vi "VITree.vi"   [LabVIEW 2016, in "DronaTest.lvlib"]
uses:
  DronaTest.lvlib
  APIs/Stimulus/ControlValue/typedef/Name&Occurrence.ctl
  APIs/Assert/AssertControlValue/AlmostEqual.vi
  APIs/Assert/AssertControlValue/Equal.vi
  APIs/Assert/AssertControlValue/NotEqual.vi
  APIs/Assert/AssertControlValue/Greater.vi
  APIs/Assert/AssertControlValue/GreaterOrEqual.vi
  APIs/Assert/AssertControlValue/Less.vi
  APIs/Assert/AssertControlValue/LessOrEqual.vi
  APIs/Assert/AssertControlValue/True.vi
  APIs/Assert/AssertControlValue/False.vi
  APIs/Assert/AssertControlDisable/AssertDisabled.vi
  APIs/Assert/AssertControlDisable/AssertDisabledAndGrayedOut.vi
  APIs/Assert/AssertControlDisable/AssertEnabled.vi
  APIs/Assert/AssertControlValue/Controls/Listbox/AssertValueByFocusIndex.vi
  APIs/Assert/AssertControlValue/Controls/Listbox/AssertValueByFocusName.vi
  APIs/Assert/AssertControlValue/Controls/Listbox/AssertValueByArrayIndex.vi
  APIs/Assert/AssertControlValue/Controls/Listbox/AssertValueByArrayName.vi
  APIs/Assert/AssertControlValue/Controls/Listbox/AssertIndexValue.vi
  APIs/Assert/AssertControlValue/Controls/Listbox/AssertAllItems.vi
  APIs/Assert/AssertControlValue/Controls/Listbox/AssertDisabledItems.vi
  APIs/Assert/AssertControlValue/Controls/MC Listbox/AssertValueByFocusIndex.vi
  APIs/Assert/AssertControlValue/Controls/MC Listbox/AssertValueByFocusName.vi
  APIs/Assert/AssertControlValue/Controls/MC Listbox/AssertValueByArrayIndex.vi
  APIs/Assert/AssertControlValue/Controls/MC Listbox/AssertValueByArrayName.vi
  APIs/Assert/AssertControlValue/Controls/MC Listbox/AssertIndexValue.vi
  APIs/Assert/AssertControlValue/Controls/MC Listbox/AssertAllItems.vi
  APIs/Assert/AssertControlValue/Controls/MC Listbox/AssertDisabledItems.vi
  APIs/Assert/AssertSubpanel/AssertSubpanelVIExecBad.vi
  APIs/Assert/AssertSubpanel/AssertSubpanelVIExecIdle.vi
  APIs/Assert/AssertSubpanel/AssertSubpanelVIExecNotBad.vi
  APIs/Assert/AssertSubpanel/AssertSubpanelVIExecRunning.vi
  APIs/Assert/AssertSubpanel/AssertSubpanelVI.vi
  APIs/Assert/AssertVI/Exec/AssertVIExecBad.vi
  APIs/Assert/AssertVI/Exec/AssertVIExecIdle.vi
  APIs/Assert/AssertVI/Exec/AssertVIExecNotBad.vi
  APIs/Assert/AssertVI/Exec/AssertVIExecRunning.vi
  APIs/Assert/AssertControlVisible/AssertVisible.vi
  APIs/Assert/AssertControlVisible/AssertInvisible.vi
  APIs/Get/GetControlValue/GetControlValueByPathString.vi
  APIs/Get/GetControlRef/GetControlRefByPath.vi
  APIs/Get/GetVI/GetVIByName.vi
  APIs/Get/GetVI/GetVIByPath.vi
  APIs/Stimulus/VI/RunVI.vi
  APIs/Stimulus/VI/OpenVIFrontPanel.vi
  APIs/Stimulus/VI/MakeVIFrontMost.vi
  APIs/Stimulus/VI/CloseVI.vi
  APIs/Stimulus/ControlValue/SetValueAuto.vi
  APIs/Stimulus/ControlValue/ValueSignalByPathString.vi
  APIs/Stimulus/ControlValue/ValueSignalLatchBooleanString.vi
  APIs/Stimulus/ControlValue/Controls/Listbox/SetValueByItemIndex.vi
  APIs/Stimulus/ControlValue/Controls/Listbox/SetValueByItemName.vi
  APIs/Stimulus/ControlValue/Controls/Listbox/SetValueByArrayIndex.vi
  APIs/Stimulus/ControlValue/Controls/Listbox/SetValueByArrayName.vi
  APIs/Stimulus/ControlValue/Controls/MC Listbox/SetValueByItemIndex.vi
  APIs/Stimulus/ControlValue/Controls/MC Listbox/SetValueByItemName.vi
  APIs/Stimulus/ControlValue/Controls/MC Listbox/SetValueByArrayIndex.vi
  APIs/Stimulus/ControlValue/Controls/MC Listbox/SetValueByArrayName.vi
  Drona.lvlib
  APIs/Get/GetVI/GetVI.lvlib
  APIs/Get/GetControlValue/GetControlValue.lvlib
  APIs/Get/GetControlRef/GetControlRef.lvlib
  APIs/Stimulus/ControlValue/ControlValue.lvlib
  APIs/Assert/AssertControlValue/AssertControlValue.lvlib
  APIs/Assert/AssertControlValue/Controls/Listbox/AssertListbox.lvlib
  APIs/Stimulus/VI/VI.lvlib
  APIs/Stimulus/ControlValue/Controls/Listbox/StimulusListbox.lvlib
  APIs/Stimulus/ControlValue/Controls/MC Listbox/StimulusMCListbox.lvlib
  APIs/Assert/AssertControlValue/Controls/MC Listbox/AssertMCListbox.lvlib
  APIs/Assert/AssertControlDisable/AssertControlDisable.lvlib
  APIs/Assert/AssertSubpanel/AssertSubpanel.lvlib
  APIs/Assert/AssertVI/AssertVI.lvlib
  AssertControlVisible.lvlib
types:
  T1 = typedef "Drona.lvlib/ControlValue.lvlib/Name&Occurrence.ctl" = cluster{"ItemName":string, "Occurrence":i32}
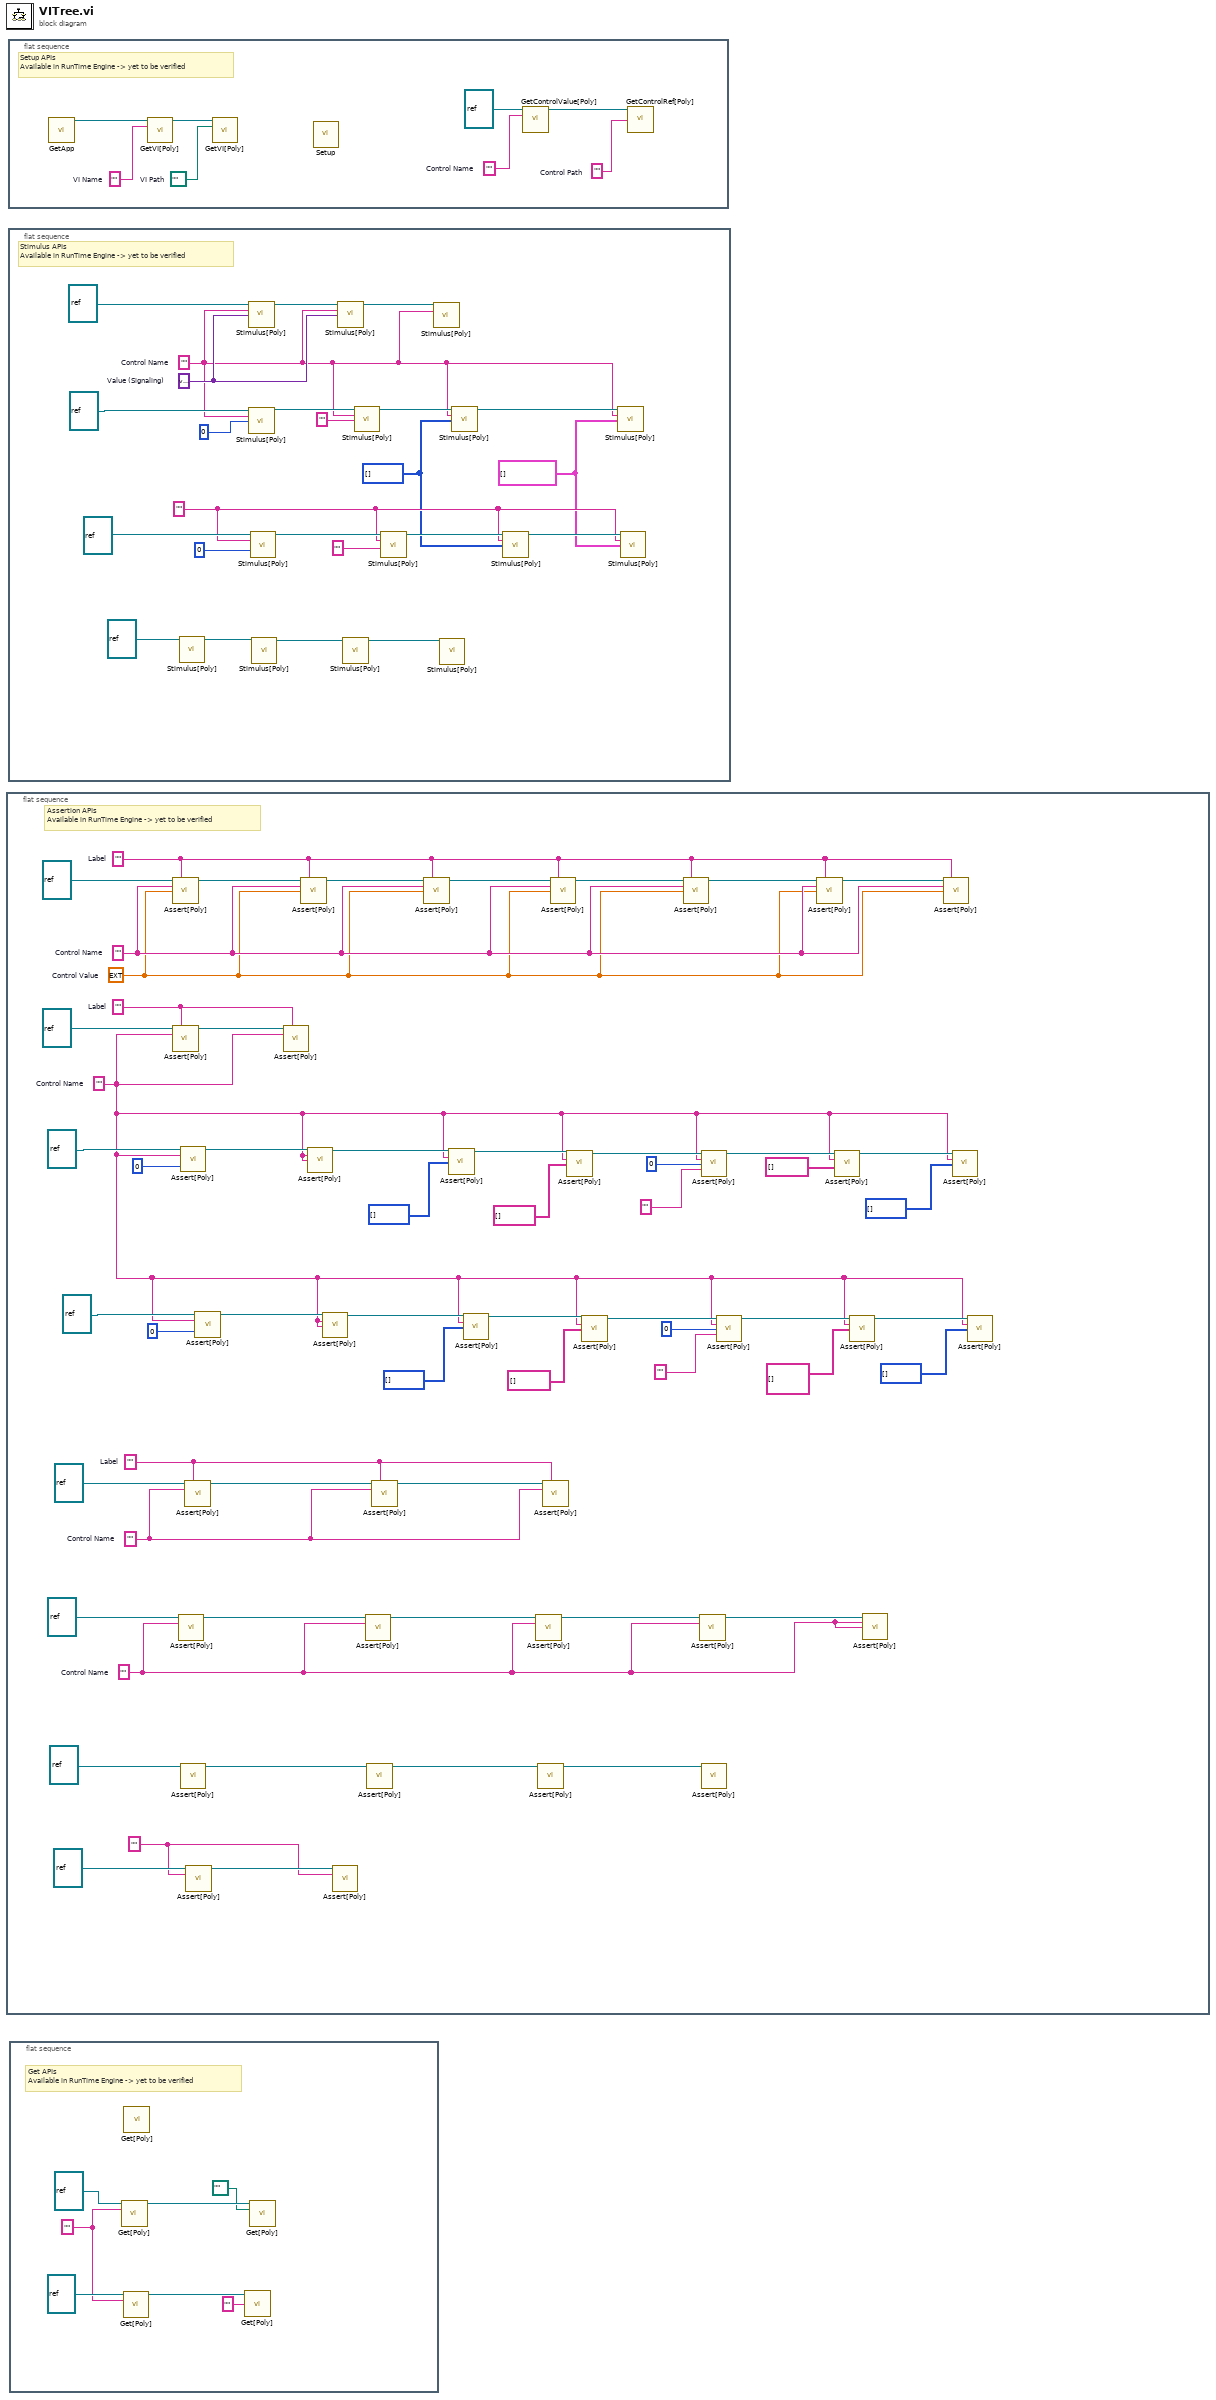
[diagram p0: block diagram]
diagram:
  n1 = flat-sequence {
    frame #0 {
      w1 = "" ("Control Path")
      w8 = ""  # Control Name
      w43 = ""  # Control Name
      w44 = ""  # Label
      w15 = ""  # Control Name
      w50 = ""  # Label
      w51 = ext 0.0  # Control Value
      w52 = ""  # Control Name
      w53 = ""  # Label
      # "Assertion APIs\nAvailable in RunTime Engine -> yet to be verified"
      n2 = call-poly "Assert[Poly].vi"("VI Reference In"=refnum<vi> refnum, "Test Label"=w53, "Control Path"=w52, "Control Value"=w51) -> ("VI Reference Out"=w59:refnum<vi>)  [unwired: 9 in, 2 out]
      n3 = call-poly "Assert[Poly].vi"("VI Reference In"=refnum<vi> refnum, "Test Label"=w50, "Control Path"=w15) -> ("VI Reference Out"=w49:refnum<vi>)  [unwired: 10 in, 2 out]
      n4 = call-poly "Assert[Poly].vi"("VI Reference In"=refnum<vi> refnum, "Control Path"=w8) -> ("VI Reference Out"=w12:refnum<vi>)  [unwired: 11 in, 2 out]
      n5 = call-poly "Assert[Poly].vi"("VI Reference In"=refnum<vi> refnum, "Control Path"=w15, "Focus Index"=0) -> ("VI Reference Out"=w41:refnum<vi>)  [unwired: 10 in, 2 out]
      n6 = call-poly "Assert[Poly].vi"("VI Reference In"=refnum<vi> refnum) -> ("VI Reference Out"=w6:refnum<vi>)  [unwired: 12 in, 2 out]
      n7 = call-poly "Assert[Poly].vi"("VI Reference In"=refnum<vi> refnum, "Test Label"=w44, "Control Path"=w43) -> ("VI Reference Out"=w46:refnum<vi>)  [unwired: 10 in, 2 out]
      n8 = call-poly "Assert[Poly].vi"("VI Reference In"=refnum<vi> refnum, "Control Path"=w1) -> ("VI Reference Out"=w3:refnum<vi>)  [unwired: 11 in, 2 out]
      n9 = call-poly "Assert[Poly].vi"("VI Reference In"=refnum<vi> refnum, "Control Path"=w15, "Focus Index"=0) -> ("VI Reference Out"=w27:refnum<vi>)  [unwired: 10 in, 2 out]
      n10 = call-poly "Assert[Poly].vi"("VI Reference In"=w49, "Test Label"=w50, "Control Path"=w15) -> ()  [unwired: 10 in, 3 out]
      n11 = call-poly "Assert[Poly].vi"("VI Reference In"=w59, "Test Label"=w53, "Control Path"=w52, "Control Value"=w51) -> ("VI Reference Out"=w58:refnum<vi>)  [unwired: 9 in, 2 out]
      n12 = call-poly "Assert[Poly].vi"("VI Reference In"=w41, "Control Path"=w15, "Item Name"=w15) -> ("VI Reference Out"=w40:refnum<vi>)  [unwired: 10 in, 2 out]
      n13 = call-poly "Assert[Poly].vi"("VI Reference In"=w27, "Control Path"=w15, "Item Name"=w15) -> ("VI Reference Out"=w26:refnum<vi>)  [unwired: 10 in, 2 out]
      n14 = call-poly "Assert[Poly].vi"("VI Reference In"=w3, "Control Path"=w1) -> ()  [unwired: 11 in, 3 out]
      n15 = call-poly "Assert[Poly].vi"("VI Reference In"=w12, "Control Path"=w8) -> ("VI Reference Out"=w11:refnum<vi>)  [unwired: 11 in, 2 out]
      n16 = call-poly "Assert[Poly].vi"("VI Reference In"=w6) -> ("VI Reference Out"=w5:refnum<vi>)  [unwired: 12 in, 2 out]
      n17 = call-poly "Assert[Poly].vi"("VI Reference In"=w46, "Test Label"=w44, "Control Path"=w43) -> ("VI Reference Out"=w45:refnum<vi>)  [unwired: 10 in, 2 out]
      n18 = call-poly "Assert[Poly].vi"("VI Reference In"=w58, "Test Label"=w53, "Control Path"=w52, "Control Value"=w51) -> ("VI Reference Out"=w57:refnum<vi>)  [unwired: 9 in, 2 out]
      n19 = call-poly "Assert[Poly].vi"("VI Reference In"=w40, "Control Path"=w15, "Focus Item Index"=i32[] []) -> ("VI Reference Out"=w39:refnum<vi>)  [unwired: 10 in, 2 out]
      n20 = call-poly "Assert[Poly].vi"("VI Reference In"=w26, "Control Path"=w15, "Focus Item Index"=i32[] []) -> ("VI Reference Out"=w25:refnum<vi>)  [unwired: 10 in, 2 out]
      n21 = call-poly "Assert[Poly].vi"("VI Reference In"=w11, "Control Path"=w8) -> ("VI Reference Out"=w10:refnum<vi>)  [unwired: 11 in, 2 out]
      n22 = call-poly "Assert[Poly].vi"("VI Reference In"=w5) -> ("VI Reference Out"=w4:refnum<vi>)  [unwired: 12 in, 2 out]
      n23 = call-poly "Assert[Poly].vi"("VI Reference In"=w45, "Test Label"=w44, "Control Path"=w43) -> ()  [unwired: 10 in, 3 out]
      n24 = call-poly "Assert[Poly].vi"("VI Reference In"=w57, "Test Label"=w53, "Control Path"=w52, "Control Value"=w51) -> ("VI Reference Out"=w56:refnum<vi>)  [unwired: 9 in, 2 out]
      n25 = call-poly "Assert[Poly].vi"("VI Reference In"=w39, "Control Path"=w15, "Focus Item Names"=string[] []) -> ("VI Reference Out"=w38:refnum<vi>)  [unwired: 10 in, 2 out]
      n26 = call-poly "Assert[Poly].vi"("VI Reference In"=w25, "Control Path"=w15, "Focus Item Names"=string[] []) -> ("VI Reference Out"=w24:refnum<vi>)  [unwired: 10 in, 2 out]
      n27 = call-poly "Assert[Poly].vi"("VI Reference In"=w56, "Test Label"=w53, "Control Path"=w52, "Control Value"=w51) -> ("VI Reference Out"=w55:refnum<vi>)  [unwired: 9 in, 2 out]
      n28 = call-poly "Assert[Poly].vi"("VI Reference In"=w10, "Control Path"=w8) -> ("VI Reference Out"=w9:refnum<vi>)  [unwired: 11 in, 2 out]
      n29 = call-poly "Assert[Poly].vi"("VI Reference In"=w38, "Control Path"=w15, "Item Index"=0, "Item Value"="") -> ("VI Reference Out"=w37:refnum<vi>)  [unwired: 9 in, 2 out]
      n30 = call-poly "Assert[Poly].vi"("VI Reference In"=w4) -> ()  [unwired: 12 in, 3 out]
      n31 = call-poly "Assert[Poly].vi"("VI Reference In"=w24, "Control Path"=w15, "Row Index"=0 ("Item Index"), "Item Value"="") -> ("VI Reference Out"=w23:refnum<vi>)  [unwired: 9 in, 2 out]
      n32 = call-poly "Assert[Poly].vi"("VI Reference In"=w55, "Test Label"=w53, "Control Path"=w52, "Control Value"=w51) -> ("VI Reference Out"=w54:refnum<vi>)  [unwired: 9 in, 2 out]
      n33 = call-poly "Assert[Poly].vi"("VI Reference In"=w37, "Control Path"=w15, "Item Names"=string[] []) -> ("VI Reference Out"=w36:refnum<vi>)  [unwired: 10 in, 2 out]
      n34 = call-poly "Assert[Poly].vi"("VI Reference In"=w23, "Control Path"=w15, "Item Names"=string[][] []) -> ("VI Reference Out"=w22:refnum<vi>)  [unwired: 10 in, 2 out]
      n35 = call-poly "Assert[Poly].vi"("VI Reference In"=w9, "Control Path"=w8, "VI Name"=w8) -> ()  [unwired: 10 in, 3 out]
      n36 = call-poly "Assert[Poly].vi"("VI Reference In"=w54, "Test Label"=w53, "Control Path"=w52, "Control Value"=w51) -> ()  [unwired: 9 in, 3 out]
      n37 = call-poly "Assert[Poly].vi"("VI Reference In"=w36, "Control Path"=w15, "Disabled Items"=i32[] []) -> ()  [unwired: 10 in, 3 out]
      n38 = call-poly "Assert[Poly].vi"("VI Reference In"=w22, "Control Path"=w15, "Disabled Items"=i32[] []) -> ()  [unwired: 10 in, 3 out]
    }
  }
  n39 = flat-sequence {
    frame #0 {
      w62 = ""  # Control Path
      w63 = ""  # Control Name
      w65 = path ""  # VI Path
      w66 = ""  # VI Name
      # "Setup APIs\nAvailable in RunTime Engine -> yet to be verified"
      n40 = call "GetApp.vi"() -> ("Application Ref"=w67:refnum<vi>)  [unwired: 14 in, 1 out]
      n41 = call-poly "GetVI[Poly].vi"("Application Ref in"=w67, "VI Name"=w66) -> ("Application Ref out"=w68:refnum<vi>)  [unwired: 11 in, 2 out]
      n42 = call-poly "GetVI[Poly].vi"("Application Ref in"=w68, "VI Path"=w65) -> ()  [unwired: 11 in, 3 out]
      n43 = call "Setup.vi"() -> ()  [unwired: 13 in, 3 out]
      n44 = call-poly "GetControlValue[Poly].vi"("VI Reference In"=refnum<vi> refnum, "Control Path"=w63) -> ("VI Reference Out"=w61:refnum<vi>)  [unwired: 11 in, 2 out]
      n45 = call-poly "GetControlRef[Poly].vi"("VI Reference In"=w61, "Control Path"=w62) -> ()  [unwired: 11 in, 3 out]
    }
  }
  n46 = flat-sequence {
    frame #0 {
      w72 = "" ("Control Path")
      w69 = T1[] [] ("Name Array")
      w70 = i32[] [] ("Index Array")
      w86 = variant  # Value (Signaling)
      w80 = ""  # Control Name
      # "Stimulus APIs\nAvailable in RunTime Engine -> yet to be verified"
      n47 = call-poly "Stimulus[Poly].vi"("VI Reference In"=refnum<vi> refnum) -> ("VI Reference Out"=w91:refnum<vi>)  [unwired: 13 in, 1 out]
      n48 = call-poly "Stimulus[Poly].vi"("VI Reference In"=refnum<vi> refnum, "Control Path"=w80, "Value (Signaling)"=w86) -> ("VI Reference Out"=w87:refnum<vi>)  [unwired: 11 in, 1 out]
      n49 = call-poly "Stimulus[Poly].vi"("VI Reference In"=refnum<vi> refnum, "Control Path"=w80, "Item Index"=0) -> ("VI Reference Out"=w83:refnum<vi>)  [unwired: 11 in, 1 out]
      n50 = call-poly "Stimulus[Poly].vi"("VI Reference In"=refnum<vi> refnum, "Control Path"=w72, "Item Index"=0) -> ("VI Reference Out"=w76:refnum<vi>)  [unwired: 11 in, 1 out]
      n51 = call-poly "Stimulus[Poly].vi"("VI Reference In"=w91) -> ("VI Reference Out"=w90:refnum<vi>)  [unwired: 13 in, 1 out]
      n52 = call-poly "Stimulus[Poly].vi"("VI Reference In"=w87, "Control Path"=w80, "Value (Signaling)"=w86) -> ("VI Reference Out"=w85:refnum<vi>)  [unwired: 11 in, 1 out]
      n53 = call-poly "Stimulus[Poly].vi"("VI Reference In"=w90) -> ("VI Reference Out"=w89:refnum<vi>)  [unwired: 13 in, 1 out]
      n54 = call-poly "Stimulus[Poly].vi"("VI Reference In"=w83, "Control Path"=w80, "Item Name"="") -> ("VI Reference Out"=w82:refnum<vi>)  [unwired: 11 in, 1 out]
      n55 = call-poly "Stimulus[Poly].vi"("VI Reference In"=w76, "Control Path"=w72, "Item Name"="") -> ("VI Reference Out"=w75:refnum<vi>)  [unwired: 11 in, 1 out]
      n56 = call-poly "Stimulus[Poly].vi"("VI Reference In"=w85, "Control Path"=w80) -> ()  [unwired: 12 in, 2 out]
      n57 = call-poly "Stimulus[Poly].vi"("VI Reference In"=w89) -> ()  [unwired: 13 in, 2 out]
      n58 = call-poly "Stimulus[Poly].vi"("VI Reference In"=w82, "Control Path"=w80, "Index Array"=w70) -> ("VI Reference Out"=w81:refnum<vi>)  [unwired: 11 in, 1 out]
      n59 = call-poly "Stimulus[Poly].vi"("VI Reference In"=w75, "Control Path"=w72, "Index Array"=w70) -> ("VI Reference Out"=w74:refnum<vi>)  [unwired: 11 in, 1 out]
      n60 = call-poly "Stimulus[Poly].vi"("VI Reference In"=w81, "Control Path"=w80, "Name Array"=w69) -> ()  [unwired: 11 in, 2 out]
      n61 = call-poly "Stimulus[Poly].vi"("VI Reference In"=w74, "Control Path"=w72, "Name Array"=w69) -> ()  [unwired: 11 in, 2 out]
    }
  }
  n62 = flat-sequence {
    frame #0 {
      w95 = "" ("VI Name")
      # "Get APIs\nAvailable in RunTime Engine -> yet to be verified"
      n63 = call-poly "Get[Poly].vi"("Application Ref in"=refnum<vi> refnum, "VI Name"=w95) -> ("Application Ref out"=w98:refnum<vi>)  [unwired: 11 in, 2 out]
      n64 = call-poly "Get[Poly].vi"("VI Reference In"=refnum<vi> refnum, "Control Path"=w95) -> ("VI Reference Out"=w94:refnum<vi>)  [unwired: 11 in, 2 out]
      n65 = call-poly "Get[Poly].vi"() -> ()  [unwired: 14 in, 2 out]
      n66 = call-poly "Get[Poly].vi"("VI Reference In"=w94, "Control Path"="") -> ()  [unwired: 11 in, 3 out]
      n67 = call-poly "Get[Poly].vi"("Application Ref in"=w98, "VI Path"=path "") -> ()  [unwired: 11 in, 3 out]
    }
  }
